vi "Close.vi"(8 "Error In":errorcluster, 11 "Audio Analyzer In":refnum<class "Audio Analyzer.lvclass">) -> (0 "Error Out":errorcluster)   [LabVIEW 2019, in "Audio Analyzer.lvclass"]
uses:
  Audio Analyzer.lvclass
  Process/Process.lvclass
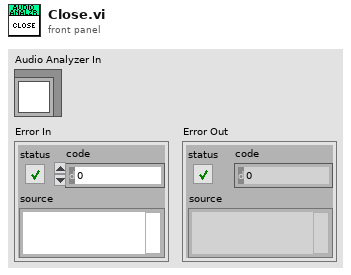
[diagram p1: front panel]
types:
  T1 = typedef "Audio Analyzer.lvclass/Data.ctl" = cluster{"Audio Spectrum Notifier":refnum<notifier>, "FPGA Reference":T2}
  T2 = typedef "Audio Analyzer.lvclass/FPGA Reference.ctl" = refnum<k20>
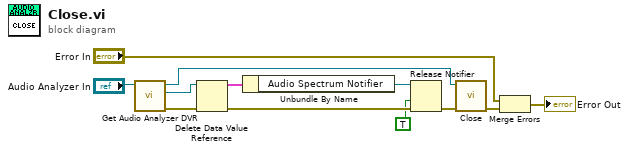
[diagram p0: block diagram]
diagram:
  n1 = call "Get Audio Analyzer DVR.vi"("Audio Analyzer In"="Audio Analyzer In") -> ("Error Out"=w9:errorcluster, "DVR"=w8:refnum<data-value>, "Audio Analyzer Out"=w10:refnum<class "Audio Analyzer.lvclass">)  [unwired: 8 in]
  n2 = Delete Data Value Reference(data value reference=w8, error in=w9) -> (data value=w7:T1, error out=w5:errorcluster)
  n3 = Unbundle By Name(w7) -> ("Audio Spectrum Notifier"=w6:refnum<notifier>)
  n4 = Release Notifier(notifier=w6, force destroy? (F)=TRUE, error in (no error)=w5) -> (error out=w3:errorcluster)  [unwired: 2 out]
  n5 = call-parent "Close.vi"("Error In"=w3, "Process In"=w10) -> ("Error Out"=w12:errorcluster)  [unwired: 9 in]
  n6 = Merge Errors("Error In", w12) -> (→"Error Out":errorcluster)
